vi "Pause.vi"(8 "error in (no error)":errorcluster, 11 "Ismatech 3 Channel Settings In":T1={"VISA resource name"="", "Pump Number"=1, "Channel Number"=0, "Simulated?"=TRUE, "Reverse?"=FALSE} {"Channel Number" min=0 max=3; "Pump Number" min=1 max=9}) -> (0 "error out":errorcluster, 1 "Connection Error":bool, 2 "5 Fails":bool, 3 "Ismatech 3 Channel Settings Out":T1={"VISA resource name"="", "Pump Number"=1, "Channel Number"=0, "Simulated?"=TRUE, "Reverse?"=FALSE} {"Channel Number" min=0 max=3; "Pump Number" min=1 max=9})   [LabVIEW 2021, in "Ismatec 4308.lvlib"]
uses:
  Ismatec 4308.lvlib
  Ismatec 4083.ctl
  support/Support Library.lvlib
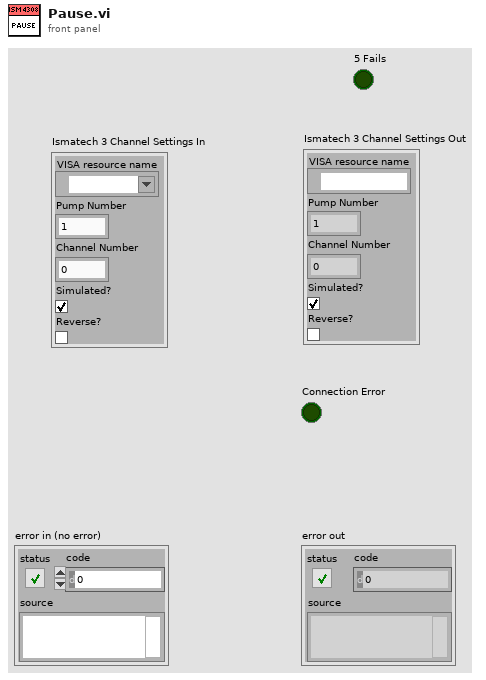
[diagram p1: front panel]
types:
  T1 = typedef "Ismatec 4308.lvlib/Ismatec 4083.ctl" = cluster{"VISA resource name":refnum<visa-resource-name>, "Pump Number":i16, "Channel Number":i16, "Simulated?":bool, "Reverse?":bool}
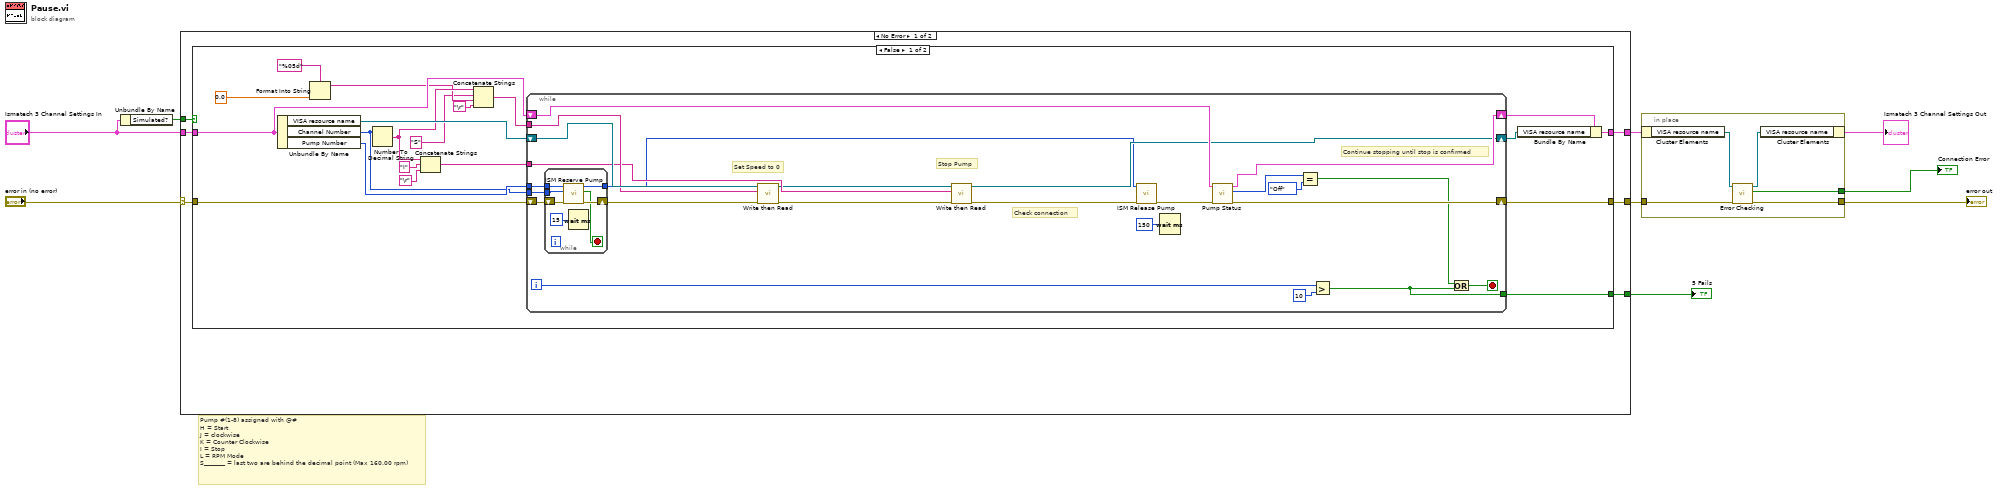
[diagram p0: block diagram]
diagram:
  # "Pump #(1-8) assigned with @#\nH = Start\nJ = clockwise\nK = Counter Clockwise\nI = Stop\nL = RPM Mode\nS_______ = last two are behind the decimal point (Max 160.00 rpm)"
  n1 = Unbundle By Name("Ismatech 3 Channel Settings In") -> ("Simulated?"=w8:bool)
  n2 = case shown="No Error" "error in (no error)" {
    selector: "error in (no error)" -> [w13 w70]
    tunnel: [w12 w69] -> w5
    tunnel: [w11 w70] -> w7
    tunnel: "Ismatech 3 Channel Settings In" -> [w15 w69]
    tunnel: w8 -> [w14 _]
    tunnel: [w10 _] -> w1
    frame No Error {
      n3 = case shown="False" w14 {
        tunnel: w15 -> [w29 w68]
        tunnel: [w35 w68] -> w12
        tunnel: w13 -> [w32 w67]
        tunnel: [w34 w67] -> w11
        tunnel: [w17 _] -> w10
        frame False {
          n4 = Unbundle By Name(w29) -> ("VISA resource name"=w31:refnum<visa-resource-name>, "Channel Number"=w16:i16, "Pump Number"=w18:i16)
          n5 = Format Into String(format string="%05d", 0.0 ("x")) -> (resulting string=w27:string)  [unwired: 2 in, 1 out]
          n6 = Number To Decimal String(number=w16) -> (decimal integer string=w30:string)  [unwired: 1 in]
          n7 = Concatenate Strings(w30, "I", "\r") -> (w19:string)
          n8 = Concatenate Strings(w30, "S" ("string"), w27, "\r") -> (w22:string)
          n9 = while {
            shift-right: [w58] -> w34
            shift-left: w32 -> [w38]
            shift-right: [w42] -> w33
            shift-left: w31 -> [w48]
            shift-right: [w56] -> w28
            shift-left: w29 -> [w57]
            tunnel: w22 -> [w47]
            tunnel: w19 -> [w45]
            tunnel: w18 -> [w40]
            tunnel: [w49] -> w17
            tunnel: w16 -> [w39]
            i -> [w52]
            stop <- w50 stop-if-true
            # "Set Speed to 0"
            # "Check connection"
            # "Stop Pump"
            # "Continue stopping until stop is confirmed"
            n10 = while {
              tunnel: w40 -> [w64]
              tunnel: w39 -> [w63]
              shift-right: [w65] -> w37
              shift-left: w38 -> [w66]
              tunnel: [w60] -> w36
              stop <- w62 stop-if-true
              n11 = call "ISM Reserve Pump.vi"("error in (no error)"=w66, "ISM Channel # In"=w63, "ISM Pump # In"=w64) -> ("error out"=w65:errorcluster, "Loop Completed"=w62:bool, "ISM Pump # Out"=w60:i32)  [unwired: 6 in]
              n12 = Wait (ms)(milliseconds to wait=u32 15) -> ()  [unwired: 1 out]
            }
            n13 = call "Write then Read.vi"("error in"=w37, "write buffer"=w47, "VISA resource name in"=w48) -> ("error out"=w46:errorcluster, "VISA resource name out"=w41:refnum<visa-resource-name>)  [unwired: 5 in, 2 out]
            n14 = call "Write then Read.vi"("error in"=w46, "write buffer"=w45, "VISA resource name in"=w41) -> ("error out"=w43:errorcluster, "VISA resource name out"=w42:refnum<visa-resource-name>)  [unwired: 5 in, 2 out]
            n15 = call "ISM Release Pump.vi"("error in (no error)"=w43, "Pump Number In"=w36) -> ("error out"=w59:errorcluster)  [unwired: 8 in, 1 out]
            n16 = Wait (ms)(milliseconds to wait=u32 150) -> ()  [unwired: 1 out]
            n17 = call "Pump Status.vi"("error in (no error)"=w59, "Ismatech 3 Channel Settings In"=w57) -> ("error out"=w58:errorcluster, "Pump On?"=w55:enum16{"Off", "On", "Not Initialized"}, "Ismatech 3 Channel Settings Out"=w56:T1)  [unwired: 5 in, 2 out]
            n18 = Equal?(x=w55, y=enum16{"Off", "On", "Not Initialized"}."Off") -> (x = y?=w53:bool)
            n19 = Greater?(x=w52, y=10) -> (0:w49:bool)
            n20 = Or(x=w53, y=w49) -> (x .or. y?=w50:bool)
          }
          n21 = Bundle By Name(cluster=w28, "VISA resource name"=w33) -> (w35:T1)
        }
        frame True {
        }
      }
    }
    frame Error {
    }
  }
  "5 Fails" <- w1
  n22 = in-place {
    in-place-border: w7 -> [w75]
    in-place-border: [w74] -> w6
    in-place-border: [w71] -> w4
    n23 = in-place-cluster #1(w5) -> ("VISA resource name"=w73:refnum<visa-resource-name>)
    n24 = call "Error Checking.vi"("error in (no error)"=w75, "VISA resource name"=w73) -> ("error out"=w71:errorcluster, "Connection Error"=w74:bool, "VISA resource name"=w72:refnum<visa-resource-name>)  [unwired: 7 in]
    n25 = in-place-cluster #1("VISA resource name"=w72) -> (→"Ismatech 3 Channel Settings Out":T1)
  }
  "Connection Error" <- w6
  "error out" <- w4
